vi "Periodic Tasks.vi"(8 "error in":errorcluster) -> ()   [LabVIEW 2015]
doc: "This VI runs in parallel to other tasks. It can contain as many user-defined periodic loops as you need. These can carry out PID or other sorts of timed response."
uses:
  <vilib>/Rock Robotics/WPI/Solenoid/WPI_SolenoidValue.ctl
  <vilib>/Rock Robotics/WPI/CAN/TalonSRX/WPI_CANTalonSRX_GlobalStatus.ctl
  <vilib>/Rock Robotics/WPI/DriverStation/WPI_DriverStationRobotMode2.ctl
  TypeDefs/estadosAutonomo.ctl
  Globales/RefNums Global.vi
  Globales/Variables Automo Global.vi
  Robot Global Data.vi
  <vilib>/Rock Robotics/WPI/Solenoid/WPI_SolenoidSetEnum.vi
  <vilib>/Rock Robotics/Network Tables/NT Read Numeric Array.vi
panel:
  out "Talon Status":T2
  in  "Talon Status":T2
  out "Distance (ft)":dbl
  in  "Catapulta Override":bool
  in  "Auto-Aim":bool
  out "Calibrated?":bool
  in  "Constante":dbl=1.0
  out "LIDAR":dbl
  in  "Value":T3=enum."Forward"
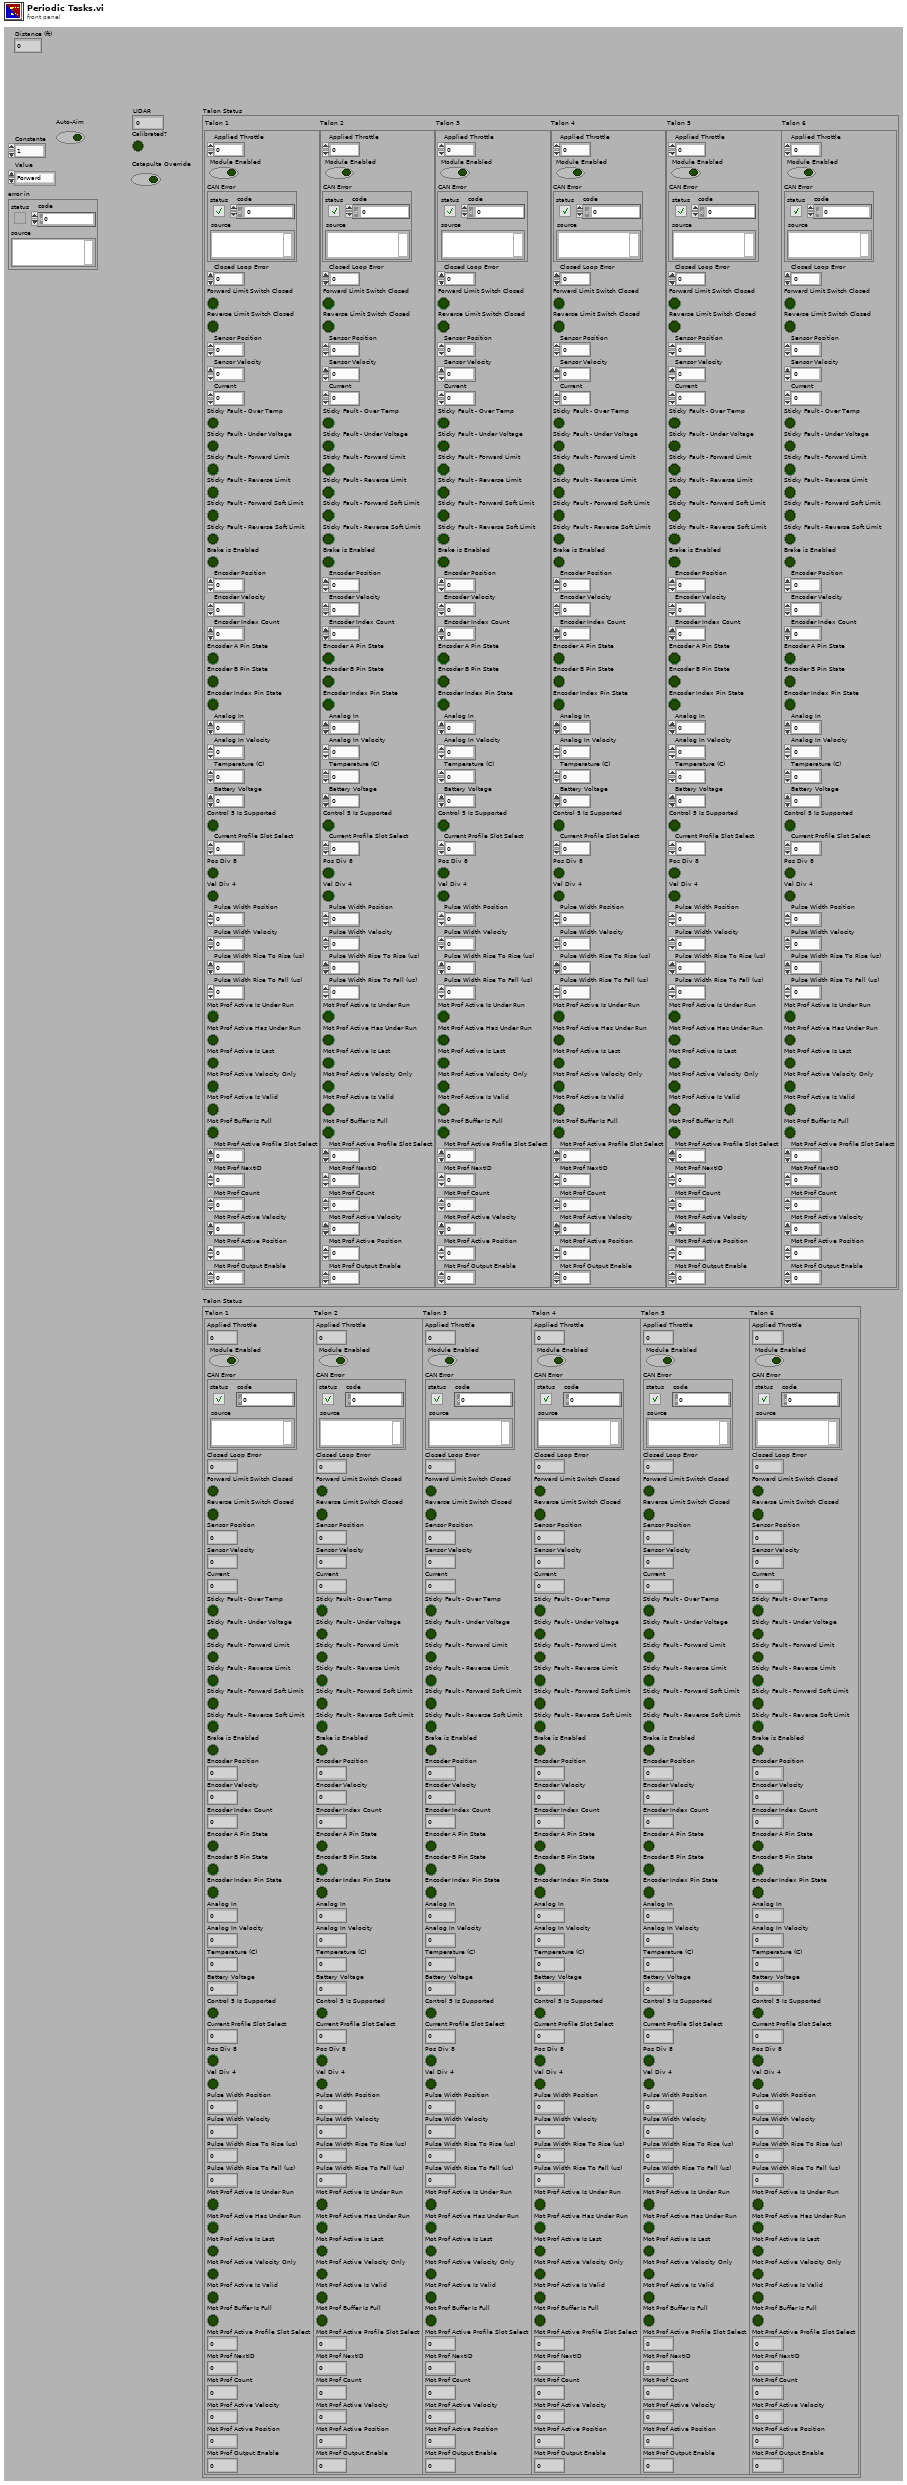
[diagram p1: front panel]
types:
  T1 = typedef "WPI_CANTalonSRX_GlobalStatus.ctl" = cluster{"Applied Throttle":dbl, "Module Enabled":bool, "CAN Error":errorcluster, "Closed Loop Error":dbl, "Forward Limit Switch Closed":bool, "Reverse Limit Switch Closed":bool, "Sensor Position":dbl, "Sensor Velocity":dbl, "Current":dbl, "Sticky Fault - Over Temp":bool, "Sticky Fault - Under Voltage":bool, "Sticky Fault - Forward Limit":bool, "Sticky Fault - Reverse Limit":bool, "Sticky Fault - Forward Soft Limit":bool, "Sticky Fault - Reverse Soft Limit":bool, "Brake is Enabled":bool, "Encoder Position":dbl, "Encoder Velocity":dbl, "Encoder Index Count":dbl, "Encoder A Pin State":bool, "Encoder B Pin State":bool, "Encoder Index Pin State":bool, "Analog In":dbl, "Analog In Velocity":dbl, "Temperature (C)":dbl, "Battery Voltage":dbl, "Control 5 Is Supported":bool, "Current Profile Slot Select":dbl, "Pos Div 8":bool, "Vel Div 4":bool, "Pulse Width Position":i32, "Pulse Width Velocity":i32, "Pulse Width Rise To Rise (us)":i32, "Pulse Width Rise To Fall (us)":i32, "Mot Prof Active Is Under Run":bool, "Mot Prof Active Has Under Run":bool, "Mot Prof Active Is Last":bool, "Mot Prof Active Velocity Only":bool, "Mot Prof Active Is Valid":bool, "Mot Prof Buffer Is Full":bool, "Mot Prof Active Profile Slot Select":i32, "Mot Prof NextID":i32, "Mot Prof Count":i32, "Mot Prof Active Velocity":dbl, "Mot Prof Active Position":dbl, "Mot Prof Output Enable":i32}
  T2 = cluster{"Talon 1":T1, "Talon 2":T1, "Talon 3":T1, "Talon 4":T1, "Talon 5":T1, "Talon 6":T1}
  T3 = typedef "WPI_SolenoidValue.ctl" = enum16{"Off", "On", "Forward", "Reverse"}
  T4 = typedef "WPI_DriverStationRobotMode2.ctl" = enum16{"Autonomous Disabled", "Autonomous Enabled", "Teleop Disabled", "Teleop Enabled", "Disconnected", "Finish", "Test Disabled", "Test Enabled", "Emergency Stopped"}
  T5 = typedef "estadosAutonomo.ctl" = enum16{"Done", "Disparar", "Auto-Aim", "Ver Torre", "Cruzar Defensa"}
  T6 = typedef "WPI_MotorControlDeviceRef.ctl" = cluster{"DeviceStatus":errorcluster, "Type":T7, "PWM":cluster{"PWM Channel":T8, "DeadBand":T9}, "CAN":cluster{"Device Number":u8, "Control Mode":T10, "Semaphore":T11, "Max Vout":dbl, "TalonSRX Control Mode":T12}, "Invert":bool}
  T7 = typedef "WPI_MotorControlType.ctl" = enum16{"PWM", "CAN", "CANTalonSRX"}
  T8 = typedef "FPGA_DIOPWMChannel.ctl" = enum8{"PWM 0", "PWM 1", "PWM 2", "PWM 3", "PWM 4", "PWM 5", "PWM 6", "PWM 7", "PWM 8", "PWM 9", "PWM MXP 0", "PWM MXP 1", "PWM MXP 2", "PWM MXP 3", "PWM MXP 4", "PWM MXP 5", "PWM MXP 6", "PWM MXP 7", "PWM MXP 8", "PWM MXP 9", "Invalid"}
  T9 = typedef "WPI_PWMDeadband.ctl" = cluster{"Name":string, "maxPositivePwm":i32, "minPositivePwm":i32, "centerPwm":i32, "maxNegativePwm":i32, "minNegativePwm":i32, "angularRange":u16}
  T10 = typedef "WPI_CANJaguar_ControlMode.ctl" = enum8{"Percent VBus", "Current", "Speed", "Position", "Voltage"}
  T11 = typedef "Semaphore RefNum" = refnum<k1>
  T12 = typedef "WPI_CANTalonSRX_APIControlMode.ctl" = enum8{"Percent VBus", "Speed", "Position", "Slave", "Unchanged / Invalid", "Voltage Compensation", "Current", "Motion Profile"}
  T13 = typedef "WPI_EncoderDevRef.ctl" = cluster{"DevStatus":errorcluster, "EncoderIndex":T14, "CounterIndex":T15, "DistancePerCount":dbl, "Decoding Type":T16}
  T14 = typedef "FPGA_EncoderIdx.ctl" = enum8{"Enc 0", "Enc 1", "Enc 2", "Enc 3", "Enc 4", "Enc 5", "Enc 6", "Enc 7", "Invalid"}
  T15 = typedef "FPGA_CounterCtrSystemIndex.ctl" = enum8{"Ctr 0", "Ctr 1", "Ctr 2", "Ctr 3", "Ctr 4", "Ctr 5", "Ctr 6", "Ctr 7", "Invalid"}
  T16 = typedef "WPI_EncoderType.ctl" = enum16{"1x", "2x", "4x"}
  T17 = typedef "WPI_SolenoidDevRef.ctl" = cluster{"DevStatus":errorcluster, "Pneumatics Control Module":u8, "Forward Solenoid Channel":T18, "Reverse Solenoid Channel":T18}
  T18 = typedef "WPI_SolenoidChannel.ctl" = enum8{"Solenoid 0", "Solenoid 1", "Solenoid 2", "Solenoid 3", "Solenoid 4", "Solenoid 5", "Solenoid 6", "Solenoid 7", "Invalid"}
  T19 = typedef "WPI_SwitchDevRef.ctl" = cluster{"DevStatus":errorcluster, "DIO Channel":T20, "CntIndex":T15, "Normally Closed":bool}
  T20 = typedef "FPGA_DIOChannel.ctl" = enum8{"DIO 0", "DIO 1", "DIO 2", "DIO 3", "DIO 4", "DIO 5", "DIO 6", "DIO 7", "DIO 8", "DIO 9", "DIO MXP 0", "DIO MXP 1", "DIO MXP 2", "DIO MXP 3", "DIO MXP 4", "DIO MXP 5", "DIO MXP 6", "DIO MXP 7", "DIO MXP 8", "DIO MXP 9", "DIO MXP 10", "DIO MXP 11", "DIO MXP 12", "DIO MXP 13", "DIO MXP 14", "DIO MXP 15", "Invalid"}
  T21 = typedef "WPI_JoystickDevRef.ctl" = cluster{"Device":T22}
  T22 = typedef "WPI_JoystickDeviceEnum.ctl" = enum16{"USB 0", "USB 1", "USB 2", "USB 3", "USB 4", "USB 5"}
  T23 = typedef "WPI_GyroDevRef.ctl" = cluster{"DevStatus":errorcluster, "Analog Channel":T24, "Offset":dbl, "Gain (VoltsPerDegree/Second)":dbl, "Gyro Type":enum16{"Analog", "XRS450"}, "Handle":i32, "SPI Bus":T25, "Device Found":bool, "Sample Rate":dbl, "Calibrate On Open":bool}
  T24 = typedef "FPGA_AIChannel.ctl" = enum8{"AI 0", "AI 1", "AI 2", "AI 3", "AI MXP 0", "AI MXP 1", "AI MXP 2", "AI MXP 3", "Invalid"}
  T25 = typedef "spi_bus.ctl" = enum16{"SPI On-Board, CS0", "SPI On-Board, CS1", "SPI On-Board, CS2", "SPI On-Board, CS3", "SPI MXP", "Invalid"}
  T26 = cluster{"Izquierda 1":T6, "Izquierda 2":T6, "Izquierda 3":T6, "Derecha 1":T6, "Derecha 2":T6, "Derecha 3":T6, "Encoder 1":T13, "Encoder 2":T13, "Feeder":T6, "Catapulta":T6, "Escalador":T6, "Largo":T17, "Corto":T17, "Cambio":T17, "Escalador":T17, "Encoder 3":T13, "Limit Catapulta":T19, "JoystickDevRef":T21, "Gyro":T23}
  T27 = cluster{"Buttons[0]":bool, "Buttons[1]":bool, "Buttons[2]":bool, "Buttons[3]":bool, "Buttons[4]":bool, "Buttons[5]":bool, "Buttons[6]":bool, "Buttons[7]":bool, "Buttons[8]":bool}
  T28 = typedef "WPI_I2CDevRef.ctl" = cluster{"DevStatus":errorcluster, "Device Address":u8, "Handle":i32, "I2C Bus":T29}
  T29 = typedef "i2c_bus.ctl" = enum16{"I2C On-Board", "I2C MXP", "Invalid"}
  T30 = cluster{"Axes[0]":dbl, "Axes[1]":dbl, "Axes[2]":dbl, "Axes[3]":dbl, "Axes[4]":dbl, "Axes[5]":dbl, "Axes[6]":dbl, "Axes[7]":dbl, "Axes[8]":dbl}
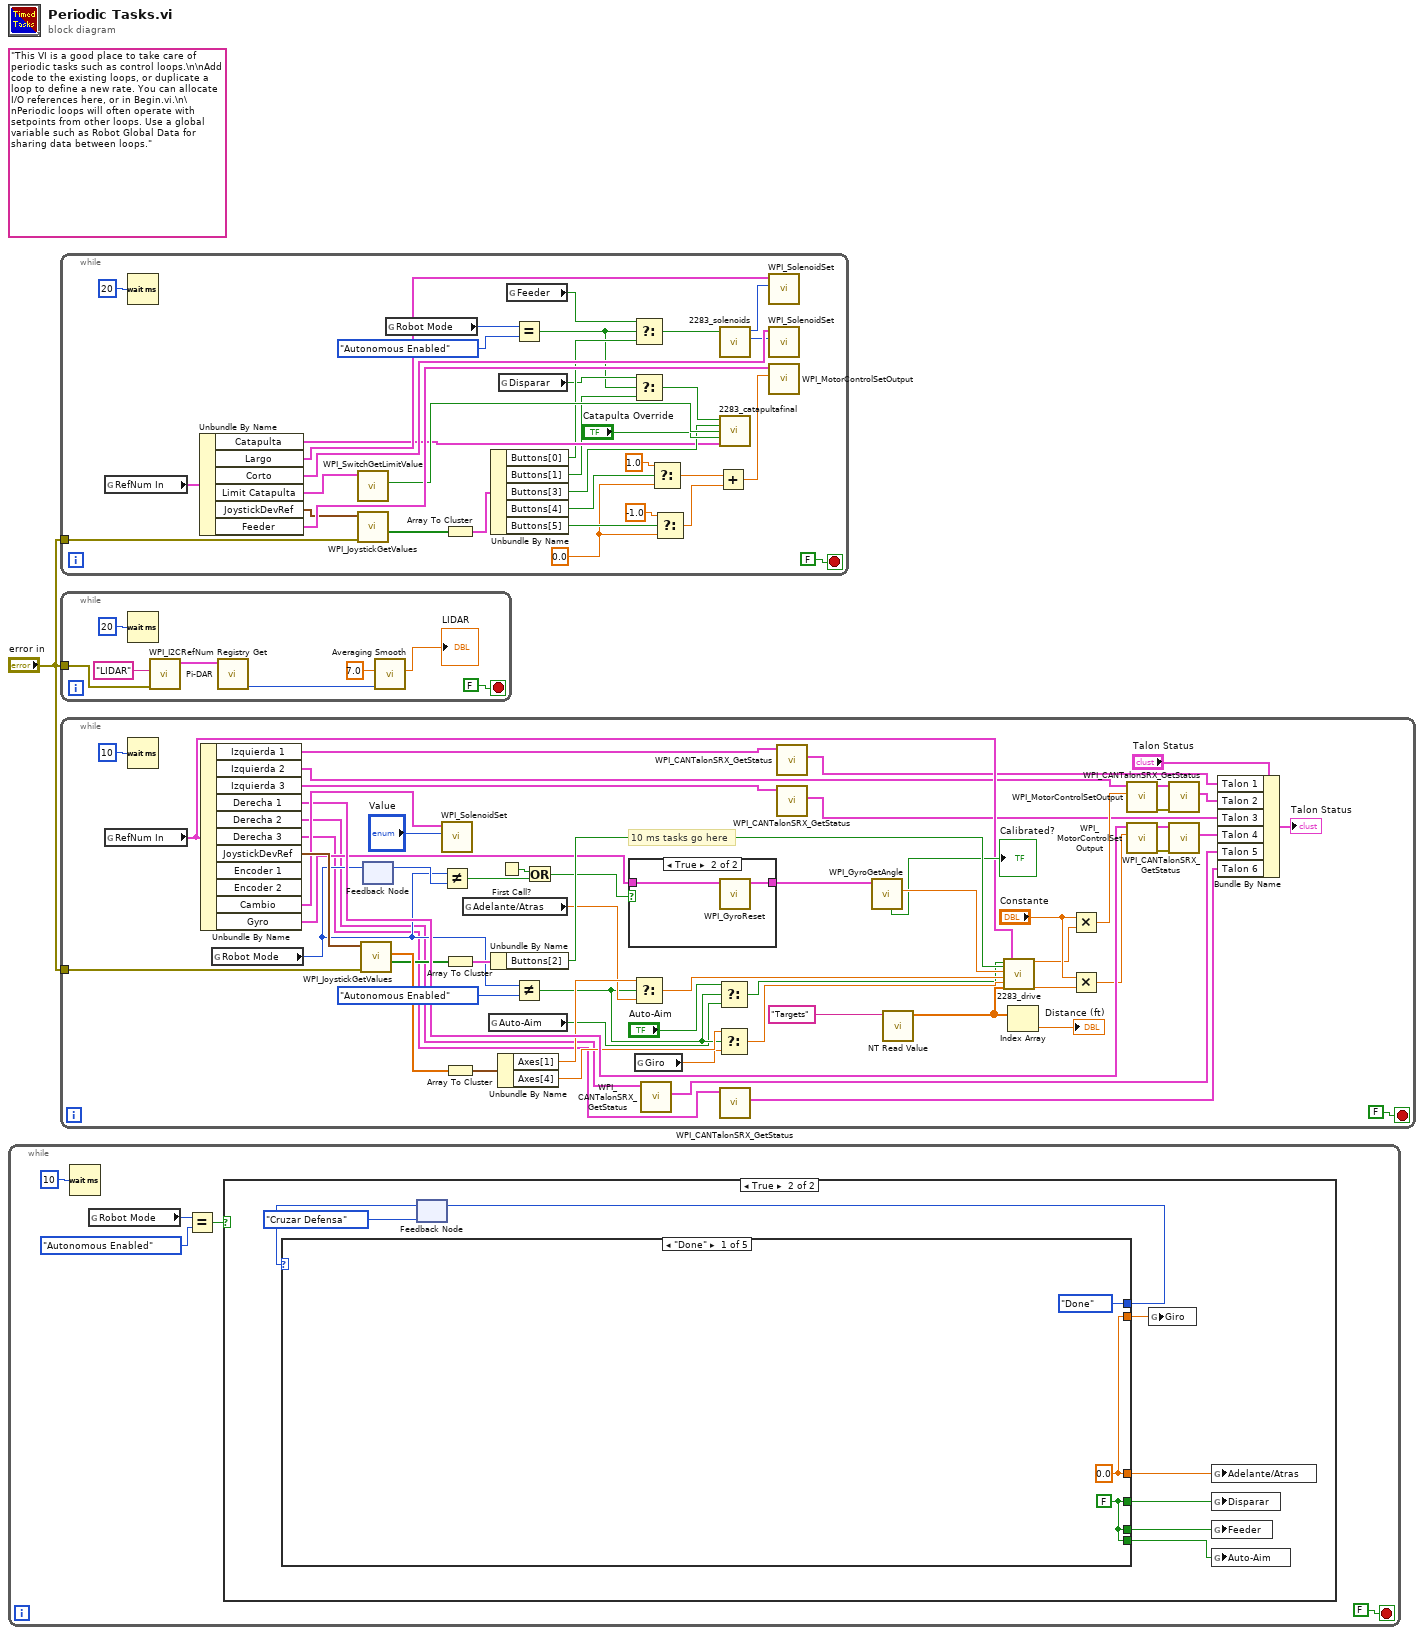
[diagram p0: block diagram]
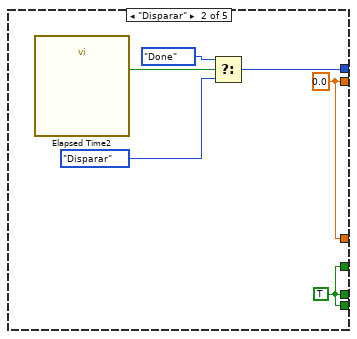
[diagram p3: hidden frame]
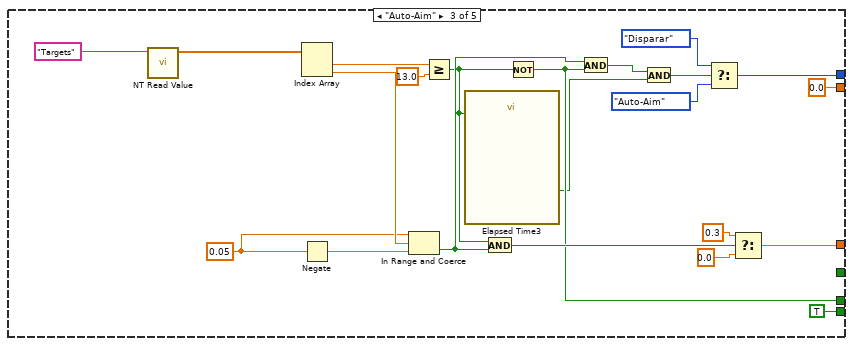
[diagram p4: hidden frame]
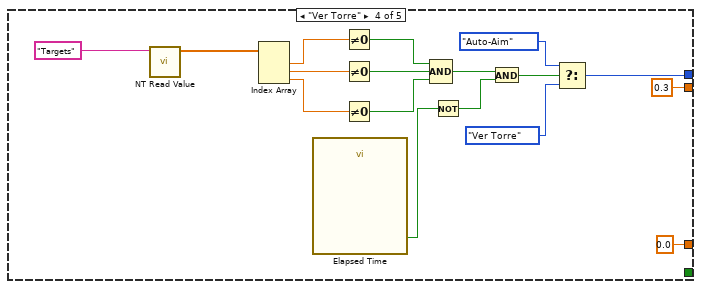
[diagram p5: hidden frame]
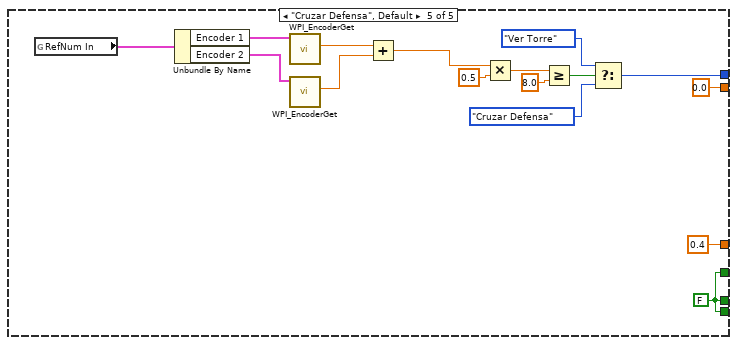
[diagram p6: hidden frame]
diagram:
  (unwired) "This VI is a good place to take care of periodic tasks such as control loops.\n\nAdd code to the existing loops, or duplicate a loop to define a new rate. You can allocate I/O references here, or in Begin.vi.\n\nPeriodic loops will often operate with setpoints from other loops. Use a global variable such as Robot Global Data for sharing data between loops."
  n1 = while {
    stop <- FALSE stop-if-true
    n2 = Wait (ms)(milliseconds to wait=u32 10) -> ()  [unwired: 1 out]
    n3 = global read "Robot Global Data.vi" "Robot Mode"() -> (w6:T4)
    n4 = Equal?(x=w6, y=WPI_DriverStationRobotMode2."Autonomous Enabled" ("Robot Mode")) -> (x = y?=w4:bool)
    n5 = case shown="True" w4 {
      frame False {
      }
      frame True {
        n6 = feedback #1(estadosAutonomo."Cruzar Defensa") -> (w13:T5)
        n7 = case shown="\"Done\"" w13 {
          tunnel: [estadosAutonomo."Done" w21 w30 w48 w78] -> w14
          tunnel: [w16 w20 w33 0.0 0.4] -> w11
          tunnel: [w16 w20 0.0 0.3 0.0] -> w10
          tunnel: [w15 w19 _ _ w63] -> w9
          tunnel: [w15 w19 w28 _ w63] -> w8
          tunnel: [w15 w19 TRUE _ w63] -> w7
          frame "Done" {
            w15 = FALSE
            w16 = 0.0 ("f")
          }
          frame "Disparar" {
            w20 = 0.0
            w19 = TRUE
            n8 = call "Elapsed Time2"() -> ("Time has Elapsed"=w18:bool)  [unwired: 12 in, 7 out]
            n9 = Select(t=estadosAutonomo."Done", s=w18, f=estadosAutonomo."Disparar") -> (s? t:f=w21:T5)
          }
          frame "Auto-Aim" {
            w37 = 0.05 ("upper limit")
            n10 = call-poly <vilib>:"NT Read Value.vi"("Name"="Targets") -> ("Numeric Array"=w42:dbl[])  [unwired: 9 in, 1 out]
            n11 = Index Array(array=w42) -> (element #1=w41:dbl, element #2=w39:dbl)  [unwired: 2 in]
            n12 = Negate(x=w37) -> (-x=w38:dbl)
            n13 = In Range and Coerce(upper limit=w37, x=w39, lower limit=w38) -> (In Range?=w29:bool)  [unwired: 1 out]
            n14 = Greater Or Equal?(x=w41, y=13.0) -> (x >= y?=w27:bool)
            n15 = call "Elapsed Time3"("Reset"=w27) -> ("Time has Elapsed"=w24:bool)  [unwired: 11 in, 7 out]
            n16 = And(x=w27, y=w29) -> (x .and. y?=w36:bool)
            n17 = Not(x=w27) -> (.not. x?=w28:bool)
            n18 = And(x=w29, y=w28) -> (x .and. y?=w25:bool)
            n19 = And(x=w25, y=w24) -> (x .and. y?=w26:bool)
            n20 = Select(t=estadosAutonomo."Disparar", s=w26, f=estadosAutonomo."Auto-Aim") -> (s? t:f=w30:T5)
            n21 = Select(t=0.3, s=w36, f=0.0) -> (s? t:f=w33:dbl)
          }
          frame "Ver Torre" {
            n22 = call-poly <vilib>:"NT Read Value.vi"("Name"="Targets") -> ("Numeric Array"=w61:dbl[])  [unwired: 9 in, 1 out]
            n23 = Index Array(array=w61) -> (element #1=w60:dbl, element #2=w59:dbl, element #3=w58:dbl)  [unwired: 3 in]
            n24 = call "Elapsed Time"() -> ("Time has Elapsed"=w52:bool)  [unwired: 12 in, 7 out]
            n25 = Not Equal To 0?(x=w60) -> (x != 0?=w57:bool)
            n26 = Not Equal To 0?(x=w59) -> (x != 0?=w56:bool)
            n27 = Not Equal To 0?(x=w58) -> (x != 0?=w55:bool)
            n28 = Compound Arithmetic op=AND(w57, w56, w55) -> (w54:bool)
            n29 = Not(x=w52) -> (.not. x?=w53:bool)
            n30 = And(x=w54, y=w53) -> (x .and. y?=w49:bool)
            n31 = Select(t=estadosAutonomo."Auto-Aim", s=w49, f=estadosAutonomo."Ver Torre") -> (s? t:f=w48:T5)
          }
          frame "Cruzar Defensa", Default {
            w63 = FALSE
            n32 = global read "RefNums Global.vi" "RefNum In"() -> (w71:T26)
            n33 = Unbundle By Name(w71) -> ("Encoder 1"=w73:T13, "Encoder 2"=w72:T13)
            n34 = call <vilib>:"WPI_EncoderGet.vi"("EncoderDevRef"=w73) -> ("Distance"=w69:dbl)  [unwired: 5 in, 5 out]
            n35 = call <vilib>:"WPI_EncoderGet.vi"("EncoderDevRef"=w72) -> ("Distance"=w70:dbl)  [unwired: 5 in, 5 out]
            n36 = Add(x=w69, y=w70) -> (x+y=w68:dbl)
            n37 = Multiply(x=w68, y=0.5) -> (x*y=w66:dbl)
            n38 = Greater Or Equal?(x=w66, y=8.0) -> (x >= y?=w65:bool)
            n39 = Select(t=estadosAutonomo."Ver Torre", s=w65, f=estadosAutonomo."Cruzar Defensa") -> (s? t:f=w78:T5)
          }
        }
        n40 = feedback-in #1(w14) -> ()
        n41 = global write "Variables Automo Global.vi" "Giro"(w10) -> ()
        n42 = global write "Variables Automo Global.vi" "Adelante/Atras"(w11) -> ()
        n43 = global write "Variables Automo Global.vi" "Disparar"(w9) -> ()
        n44 = global write "Variables Automo Global.vi" "Feeder"(w8) -> ()
        n45 = global write "Variables Automo Global.vi" "Auto-Aim"(w7) -> ()
      }
    }
  }
  n46 = while {
    tunnel: "error in" -> [w89]
    stop <- FALSE stop-if-true
    w102 = 0.0 ("f")
    n47 = global read "RefNums Global.vi" "RefNum In"() -> (w112:T26)
    n48 = Wait (ms)(milliseconds to wait=u32 20) -> ()  [unwired: 1 out]
    n49 = Unbundle By Name(w112) -> ("Catapulta"=w88:T6, "Largo"=w111:T17, "Corto"=w110:T17, "Limit Catapulta"=w109:T19, "JoystickDevRef"=w93:T21, "Feeder"=w105:T6)
    n50 = call <vilib>:"WPI_SwitchGetLimitValue.vi"("SwitchDevRef"=w109) -> ("Switch Pressed"=w96:bool)  [unwired: 8 in, 2 out]
    n51 = call <vilib>:"WPI_JoystickGetValues.vi"("error in (no error)"=w89, "JoystickDevRef"=w93) -> ("Buttons"=w92:bool[])  [unwired: 5 in, 4 out]
    n52 = global read "Robot Global Data.vi" "Robot Mode"() -> (w86:T4)
    n53 = Array To Cluster(array=w92) -> (cluster=w108:T27)
    n54 = Unbundle By Name(w108) -> ("Buttons[0]"=w84:bool, "Buttons[1]"=w81:bool, "Buttons[3]"=w94:bool, "Buttons[4]"=w104:bool, "Buttons[5]"=w103:bool)
    n55 = global read "Variables Automo Global.vi" "Disparar"() -> (w80:bool)
    n56 = global read "Variables Automo Global.vi" "Feeder"() -> (w83:bool)
    n57 = Equal?(x=w86, y=WPI_DriverStationRobotMode2."Autonomous Enabled" ("Robot Mode")) -> (x = y?=w79:bool)
    n58 = Select(t=w83, s=w79, f=w84) -> (s? t:f=w85:bool)
    n59 = Select(t=w80, s=w79, f=w81) -> (s? t:f=w82:bool)
    n60 = Select(t=1.0, s=w104, f=w102) -> (s? t:f=w99:dbl)
    n61 = Select(t=-1.0, s=w103, f=w102) -> (s? t:f=w100:dbl)
    n62 = Add(x=w99, y=w100) -> (x+y=w98:dbl)
    n63 = call "2283_solenoids.vi"("feeder"=w85) -> ("solenoidCorto"=w106:T3, "solenoidLargo"=w107:T3)  [unwired: 9 in]
    n64 = call "2283_catapultafinal.vi"("catapulta"=w82, "Reset"=w94, "swithLimit"=w96, "cargar en pits"="Catapulta Override", "CAN Talon SRX Ref"=w88) -> ()  [unwired: 11 in]
    n65 = call-poly <vilib>:"WPI_SolenoidSet.vi"("Value"=w107, "SolenoidDevRef"=w111) -> ()  [unwired: 8 in, 2 out]
    n66 = call-poly <vilib>:"WPI_SolenoidSet.vi"("Value"=w106, "SolenoidDevRef"=w110) -> ()  [unwired: 8 in, 2 out]
    n67 = call <vilib>:"WPI_MotorControlSetOutput.vi"("Output"=w98, "MotorControlDevRef"=w105) -> ()  [unwired: 7 in, 3 out]
  }
  n68 = while {
    tunnel: "error in" -> [w113]
    stop <- FALSE stop-if-true
    n69 = Wait (ms)(milliseconds to wait=u32 20) -> ()  [unwired: 1 out]
    n70 = call <vilib>:"WPI_I2CRefNum Registry Get.vi"("error in (no error)"=w113, "refnum name"="LIDAR") -> ("I2CDevRef"=w117:T28)  [unwired: 8 in, 1 out]
    n71 = call "Pi-DAR.vi"("I2CDevRef"=w117) -> ("Distance Output"=w119:i32)  [unwired: 9 in, 1 out]
    n72 = call "Averaging Smooth.vi"("Input"=w119, "# of Samples to Average"=7.0) -> ("Output"=→"LIDAR":dbl)  [unwired: 6 in, 1 out]
  }
  n73 = while {
    tunnel: "error in" -> [w164]
    stop <- FALSE stop-if-true
    # "10 ms tasks go here"
    n74 = global read "RefNums Global.vi" "RefNum In"() -> (w149:T26)
    n75 = Wait (ms)(milliseconds to wait=u32 10) -> ()  [unwired: 1 out]
    n76 = Unbundle By Name(w149) -> ("Izquierda 1"=w130:T6, "Izquierda 2"=w133:T6, "Izquierda 3"=w129:T6, "Derecha 1"=w171:T6, "Derecha 2"=w132:T6, "Derecha 3"=w131:T6, "JoystickDevRef"=w174:T21, "Cambio"=w173:T17, "Gyro"=w156:T23)  [unwired: 2 out]
    n77 = global read "Robot Global Data.vi" "Robot Mode"() -> (w144:T4)
    n78 = call <vilib>:"WPI_JoystickGetValues.vi"("error in (no error)"=w164, "JoystickDevRef"=w174) -> ("Buttons"=w162:bool[], "Axes"=w176:dbl[])  [unwired: 5 in, 3 out]
    n79 = feedback #2() -> (w159:T4)  [unwired: 1 in]
    n80 = feedback-in #2(w144) -> ()
    n81 = call-poly <vilib>:"WPI_SolenoidSet.vi"("Value"="Value", "SolenoidDevRef"=w173) -> ()  [unwired: 8 in, 2 out]
    n82 = Not Equal?(x=w144, y=w159) -> (x != y?=w158:bool)
    n83 = Array To Cluster(array=w162) -> (cluster=w163:T27)
    n84 = Array To Cluster(array=w176) -> (cluster=w175:T30)
    n85 = global read "Variables Automo Global.vi" "Adelante/Atras"() -> (w143:dbl)
    n86 = global read "Variables Automo Global.vi" "Auto-Aim"() -> (w140:bool)
    n87 = Unbundle By Name(w163) -> ("Buttons[2]"=w161:bool)
    n88 = First Call?() -> (First Call?: T/F=w160:bool)
    n89 = Unbundle By Name(w175) -> ("Axes[1]"=w146:dbl, "Axes[4]"=w165:dbl)
    n90 = Not Equal?(x=w144, y=WPI_DriverStationRobotMode2."Autonomous Enabled" ("Robot Mode")) -> (x != y?=w141:bool)
    n91 = Or(x=w160, y=w158) -> (x .or. y?=w157:bool)
    n92 = case shown="True" w157 {
      tunnel: w156 -> [w179 w181]
      tunnel: [w179 w180] -> w155
      frame False {
      }
      frame True {
        n93 = call <vilib>:"WPI_GyroReset.vi"("GyroDevRef"=w181) -> ("GyroDevRef"=w180:T23)  [unwired: 9 in, 1 out]
      }
    }
    n94 = Select(t=w146, s=w141, f=w143) -> (s? t:f=w147:dbl)
    n95 = global read "Variables Automo Global.vi" "Giro"() -> (w142:dbl)
    n96 = call <vilib>:"WPI_CANTalonSRX_GetStatus.vi"("CAN Talon SRX Ref"=w132) -> ("Talon SRX Status"=w122:T1)  [unwired: 8 in, 2 out]
    n97 = Select(t="Auto-Aim", s=w141, f=w140) -> (s? t:f=w138:bool)
    n98 = Select(t=w165, s=w141, f=w142) -> (s? t:f=w148:dbl)
    n99 = call <vilib>:"WPI_CANTalonSRX_GetStatus.vi"("CAN Talon SRX Ref"=w131) -> ("Talon SRX Status"=w121:T1)  [unwired: 8 in, 2 out]
    n100 = call <vilib>:"WPI_CANTalonSRX_GetStatus.vi"("CAN Talon SRX Ref"=w130) -> ("Talon SRX Status"=w126:T1)  [unwired: 8 in, 2 out]
    n101 = call <vilib>:"WPI_CANTalonSRX_GetStatus.vi"("CAN Talon SRX Ref"=w129) -> ("Talon SRX Status"=w125:T1)  [unwired: 8 in, 2 out]
    n102 = call <vilib>:"WPI_GyroGetAngle.vi"("GyroDevRef"=w155) -> ("Angle"=w154:dbl, "Calibrated?"=→"Calibrated?":bool)  [unwired: 6 in, 3 out]
    n103 = call-poly <vilib>:"NT Read Value.vi"("Name"="Targets") -> ("Numeric Array"=w152:dbl[])  [unwired: 9 in, 1 out]
    n104 = call "2283_drive.vi"("Auto-Aim"=w138, "Invert"=w161, "Gyro Angle"=w154, "Axes[1]"=w147, "Axis[4]"=w148, "Numeric Array"=w152, "RefNum In"=w149) -> ("Motor Izquierdo"=w167:dbl, "Motor Derecho"=w166:dbl)  [unwired: 11 in]
    n105 = Index Array(array=w152) -> (element=→"Distance (ft)":dbl)  [unwired: 1 in]
    n106 = Multiply(x="Constante", y=w167) -> (x*y=w170:dbl)
    n107 = Multiply(x="Constante", y=w166) -> (x*y=w168:dbl)
    n108 = call <vilib>:"WPI_MotorControlSetOutput.vi"("Output"=w170, "MotorControlDevRef"=w133) -> ("error out"=w137:errorcluster, "MotorControlDevRef"=w136:T6)  [unwired: 7 in, 1 out]
    n109 = call <vilib>:"WPI_MotorControlSetOutput.vi"("Output"=w168, "MotorControlDevRef"=w171) -> ("error out"=w134:errorcluster, "MotorControlDevRef"=w135:T6)  [unwired: 7 in, 1 out]
    n110 = call <vilib>:"WPI_CANTalonSRX_GetStatus.vi"("error in (no error)"=w137, "CAN Talon SRX Ref"=w136) -> ("Talon SRX Status"=w124:T1)  [unwired: 7 in, 2 out]
    n111 = call <vilib>:"WPI_CANTalonSRX_GetStatus.vi"("error in (no error)"=w134, "CAN Talon SRX Ref"=w135) -> ("Talon SRX Status"=w123:T1)  [unwired: 7 in, 2 out]
    n112 = Bundle By Name(cluster="Talon Status", "Talon 1"=w126, "Talon 2"=w124, "Talon 3"=w125, "Talon 4"=w123, "Talon 5"=w122, "Talon 6"=w121) -> (→"Talon Status":T2)
  }
